vi "Send Move Command.vi"(3 "ConnectArray IN":T4(array[cluster]), 4 "client name":string, 5 "CamConfig":T2={"ID"=0.0, "Name"="", "DeviceID"={"Slot Connector"=0, "IP Adress"="", "Port"=0, "Type"=""}, "CorrectConfig Cluster"={"Detection Parameters"={"Contrast"=0, "Treshold"=0, "Max Intensity"=0, "Max Intensity%"=0, "Rx"=0, "Ry"=0, "R%"=0.0}, "Reverse"={"Reverse X"=FALSE, "Reverse Y"=FALSE}, "Target"={"X Target"=0.0, "Y Target"=0.0}, "Region of Interest"=[-1, -1, 32000, 32000], "Correction Parameters"={"X"=5.0, "Y"=5.0, "Movement Type"=0}, "Acquisition Parameters"={"Brightness"=0.0, "Contrast"=1.0, "Saturation"=1.0, "White level"=0.7}, "Background Path"=path "", "Reference Path"=path "", "XCalibration"=[], "YCalibration"=[]}, "Ontrak Channel"=0, "IMAQdx Session 2"="cam2", "ImageServer"={"IPAddress"="", "Port"=0}} {"CorrectConfig Cluster"."Acquisition Parameters"."White level" scale=0.3..1.26 scale format="%#_2f"; "CorrectConfig Cluster"."Acquisition Parameters"."Saturation" scale=0.5..1.5 scale format="%#_3f"; "CorrectConfig Cluster"."Acquisition Parameters"."Contrast" scale=0.4..1.5 scale format="%#_3f"; "CorrectConfig Cluster"."Acquisition Parameters"."Brightness" scale=-50.0..50.0 scale format="%#_2f"; "CorrectConfig Cluster"."Correction Parameters"."Movement Type" items=["Step", "Proportionnal"]; "CorrectConfig Cluster"."Target"."X Target" format="%#_5g"; "CorrectConfig Cluster"."Target"."Y Target" format="%#_5g"; "CorrectConfig Cluster"."Detection Parameters"."Max Intensity%" max=100 step=1}, 6 "Move XY":T3(array[cluster])) -> (0 "ConnectArray Out":T4(array[cluster])=[{"IPaddress"="127.0.0.1", "Port"=63400, "connection ID"=refnum, "TCP error"={"status"=TRUE, "code"=1, "source"="TCP Write in TCPwrite8bytesMC.vi->PicoCmdClientMOVE-ForMasterControl_3.vi->Manual command_11.vi"}}], 1 "TCPconnecCmd":bool, 2 "status":string)   [LabVIEW 2013]
uses:
  <vilib>/userdefined/High Color/IMAQdx.ctl
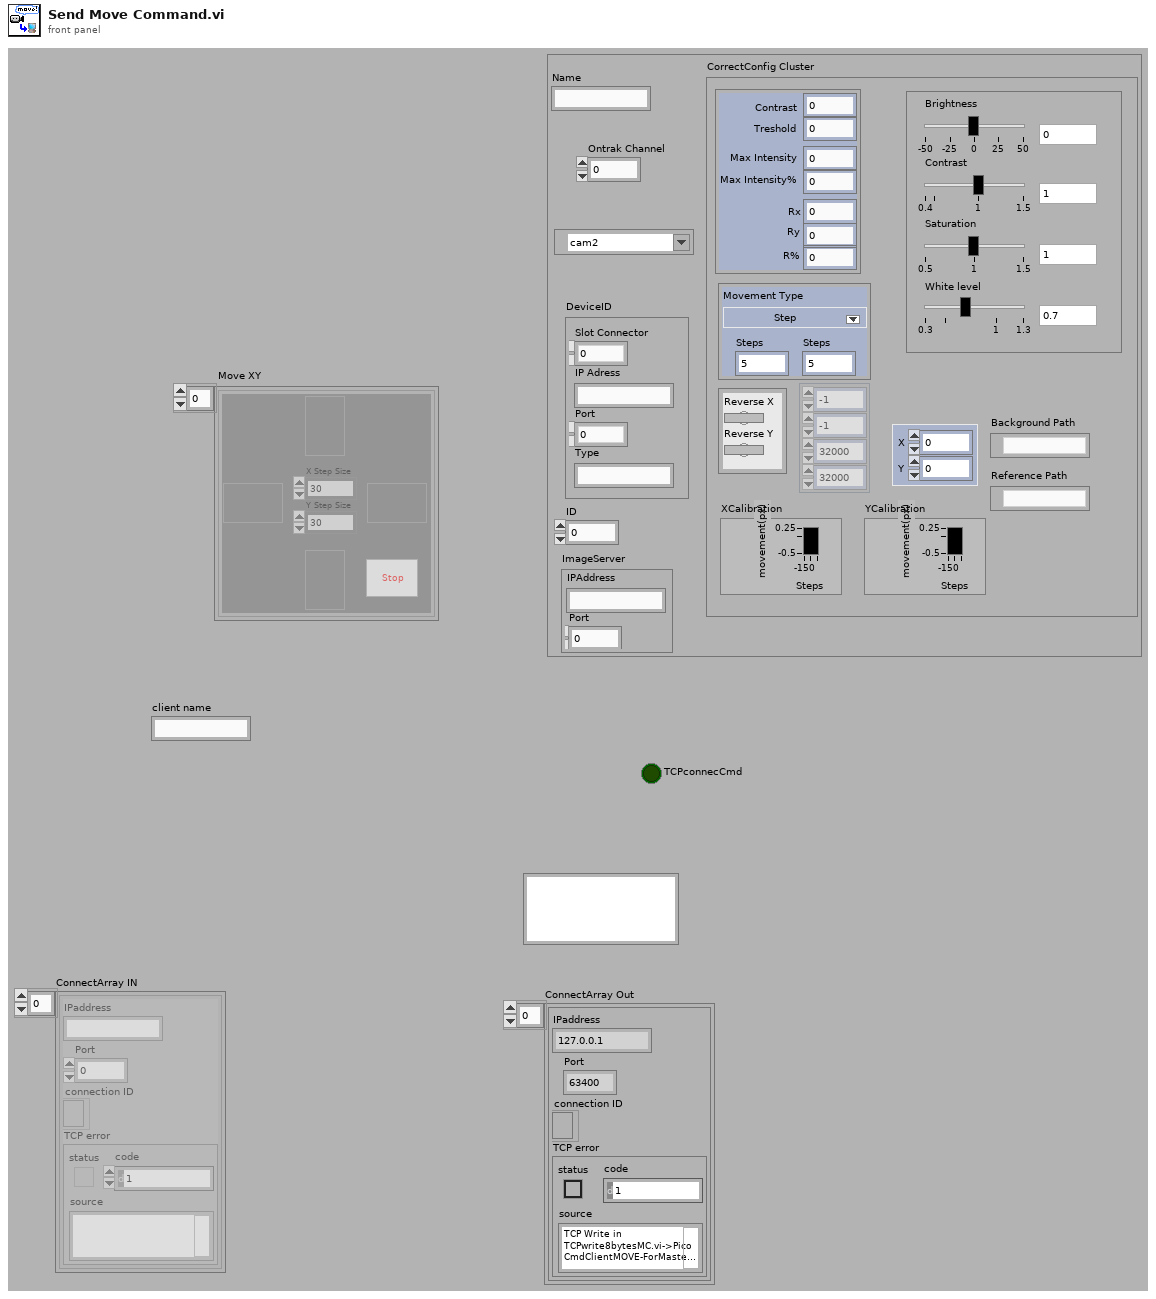
[diagram p1: front panel]
types:
  T1 = typedef "IMAQdx.ctl" = refnum<k21>
  T2 = cluster{"ID":dbl, "Name":string, "DeviceID":cluster{"Slot Connector":i32, "IP Adress":string, "Port":i32, "Type":string}, "CorrectConfig Cluster":cluster{"Detection Parameters":cluster{"Contrast":i32, "Treshold":u8, "Max Intensity":i32, "Max Intensity%":u8, "Rx":i32, "Ry":i32, "R%":sgl}, "Reverse":cluster{"Reverse X":bool, "Reverse Y":bool}, "Target":cluster{"X Target":sgl, "Y Target":sgl}, "Region of Interest":i32[], "Correction Parameters":cluster{"X":sgl, "Y":sgl, "Movement Type":u16}, "Acquisition Parameters":cluster{"Brightness":dbl, "Contrast":dbl, "Saturation":dbl, "White level":dbl}, "Background Path":path, "Reference Path":path, "XCalibration":cluster{dbl, dbl}[], "YCalibration":cluster{dbl, dbl}[]}, "Ontrak Channel":i16, "IMAQdx Session 2":T1, "ImageServer":cluster{"IPAddress":string, "Port":i32}}
  T3 = cluster{"Down":bool, "Up":bool, "Right":bool, "Left":bool, "APulses X":u16, "APulses Y":u16, "Stop":bool}[]
  T4 = cluster{"IPaddress":string, "Port":i32, "connection ID":refnum<k5>, "TCP error":errorcluster}[]
  T5 = cluster{"Slot Connector":i32, "IP Adress":string, "Port":i32, "Type":string}
  T6 = cluster{"Detection Parameters":cluster{"Contrast":i32, "Treshold":u8, "Max Intensity":i32, "Max Intensity%":u8, "Rx":i32, "Ry":i32, "R%":sgl}, "Reverse":cluster{"Reverse X":bool, "Reverse Y":bool}, "Target":cluster{"X Target":sgl, "Y Target":sgl}, "Region of Interest":i32[], "Correction Parameters":cluster{"X":sgl, "Y":sgl, "Movement Type":u16}, "Acquisition Parameters":cluster{"Brightness":dbl, "Contrast":dbl, "Saturation":dbl, "White level":dbl}, "Background Path":path, "Reference Path":path, "XCalibration":cluster{dbl, dbl}[], "YCalibration":cluster{dbl, dbl}[]}
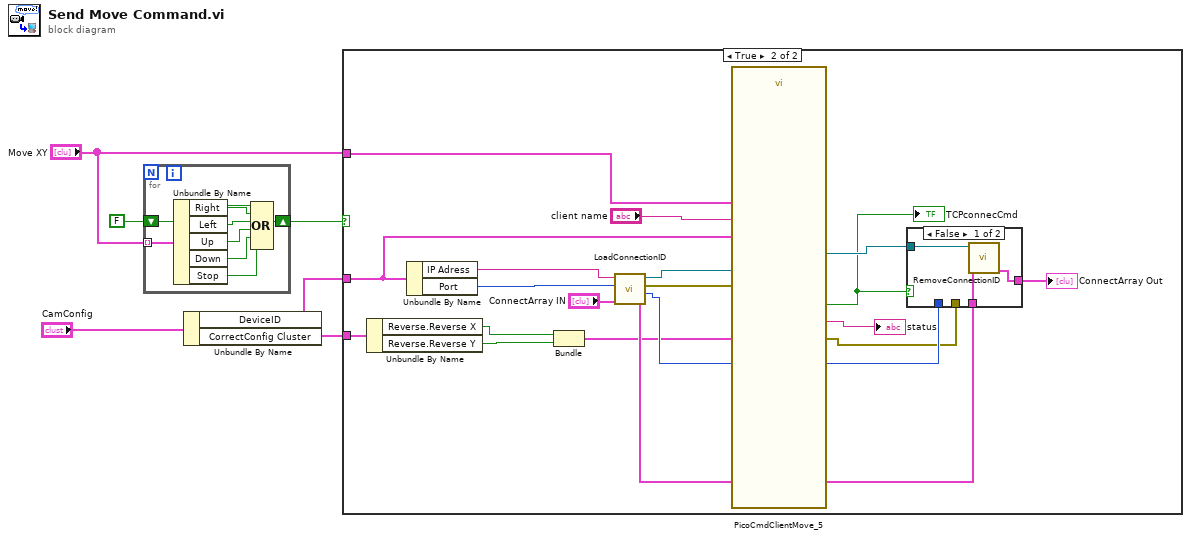
[diagram p0: block diagram]
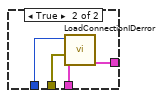
[diagram p3: hidden frame]
diagram:
  n1 = for {
    tunnel: "Move XY" -> [w14] mode=indexing
    shift-right: [w8] -> w3
    shift-left: FALSE -> [w9]
    n2 = Unbundle By Name(w14) -> ("Right"=w13:bool, "Left"=w12:bool, "Up"=w11:bool, "Down"=w10:bool, "Stop"=w7:bool)
    n3 = Compound Arithmetic op=OR(w9, w13, w12, w11, w10, w7) -> (w8:bool)
  }
  n4 = Unbundle By Name("CamConfig") -> ("DeviceID"=w6:T5, "CorrectConfig Cluster"=w5:T6)
  n5 = case shown="True" w3 {
    tunnel: w6 -> [_ w15]
    tunnel: "Move XY" -> [_ w21]
    tunnel: w5 -> [_ w20]
    frame False {
    }
    frame True {
      n6 = Unbundle By Name(w20) -> ("Reverse.Reverse X"=w19:bool, "Reverse.Reverse Y"=w18:bool)
      n7 = Unbundle By Name(w15) -> ("IP Adress"=w17:string, "Port"=w16:i32)
      n8 = Bundle("Reverse X"=w19, "Reverse Y"=w18) -> (w22:cluster{"Reverse X":bool, "Reverse Y":bool})  [unwired: 1 in]
      n9 = call "LoadConnectionID.vi"("ArrayIN"="ConnectArray IN", "Port"=w16, "IPaddress"=w17) -> ("ArrayOUT"=w33:T4, "index"=w32:i32, "ConnectError"=w31:errorcluster, "connection ID"=w30:refnum<k5>)  [unwired: 5 out]
      n10 = call "PicoCmdClientMove_5.vi"("DeviceID"=w15, "Error in"=w31, "Reverse"=w22, "Move XY"=w21, "connection ID in"=w30, "client name"="client name") -> ("connection ID out"=w28:refnum<k5>, "TCPconnectionCmd"=w26:bool, "status"=→"status":string, "error out"=w29:errorcluster)  [unwired: 18 in]
      "TCPconnecCmd" <- w26
      n11 = case shown="False" w26 {
        tunnel: w32 -> [_ w40]
        tunnel: w33 -> [w36 w39]
        tunnel: [w35 w38] -> w24
        tunnel: w29 -> [_ w37]
        tunnel: w28 -> [w34 _]
        frame False {
          n12 = call "RemoveConnectionID.vi"("ArrayIN"=w36, "connection ID"=w34) -> ("ArrayOUT"=w35:T4)  [unwired: 9 out]
        }
        frame True {
          n13 = call "LoadConnectionIDerror.vi"("ArrayIN"=w39, "ErrorIn"=w37, "index"=w40) -> ("ArrayOUT"=w38:T4)  [unwired: 8 out]
        }
      }
      "ConnectArray Out" <- w24
    }
  }
